vi "单点标定.vi"(8 "error in":errorcluster, 10 "T":i32 format="%.0x") -> (0 "error out":errorcluster, 2 "return":i32)   [LabVIEW 2016]
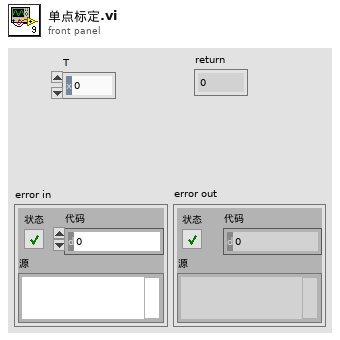
[diagram p1: front panel]
types:
  T1 = cluster{"byCmdType":u8, "bySubCmd":u8, "byPara":u8, "byAddr_h":u8, "byAddr_l":u8, "byAddr_ll":u8, "byLen_h":u8, "byLen_l":u8}
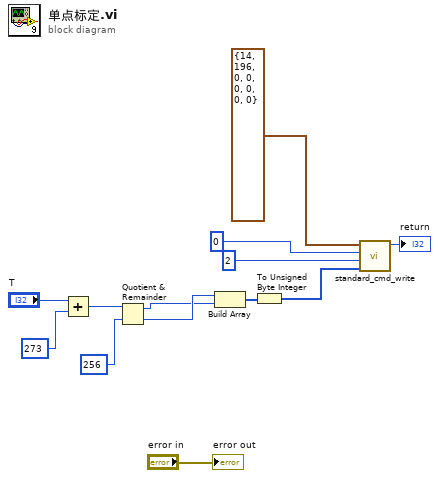
[diagram p0: block diagram]
diagram:
  n1 = Add(x="T", y=273) -> (x+y=w6:i32)
  n2 = Quotient & Remainder(x=w6, y=256) -> (x-y*floor(x/y)=w3:i32, floor(x/y)=w4:i32)
  n3 = Build Array(w4, w3) -> (w2:i32[])
  n4 = To Unsigned Byte Integer(number=w2) -> (unsigned 8bit integer=w1:u8[])
  n5 = call "standard_cmd_write.vi"("data"=w1, "dwLen"=u32 2, "dwAddr"=u32 0, "cmd_std_header_t"=T1 {"byCmdType"=14, "bySubCmd"=196, "byPara"=0, "byAddr_h"=0, "byAddr_l"=0, "byAddr_ll"=0, "byLen_h"=0, "byLen_l"=0}) -> ("return"=→"return":i32)  [unwired: 6 in, 1 out]
  "error out" <- "error in"
